vi "P3_2_Complmentos_Simulacion.vi"() -> ()   [LabVIEW 2020]
panel:
  out "consumo de lecha para chocomilk":dynamicdata(graph)
  out "m3 de leche":dbl(knob) scale=0.0..20.0
  out "valor maximo":i32
  out "dato ultimo de leche":i32
  out "calcetoce":dbl(slide) caption="Agua" scale=0.0..20.0
  out "procesos":i32
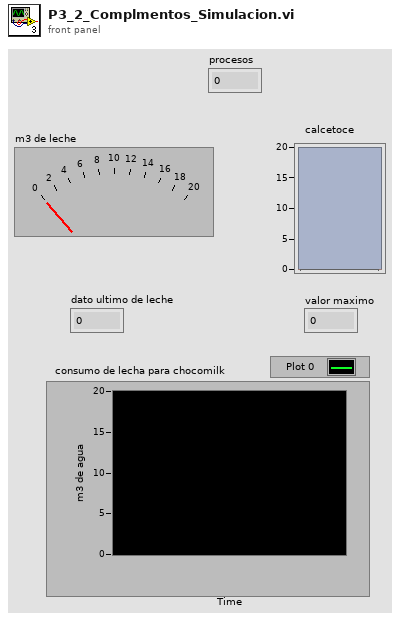
[diagram p1: front panel]
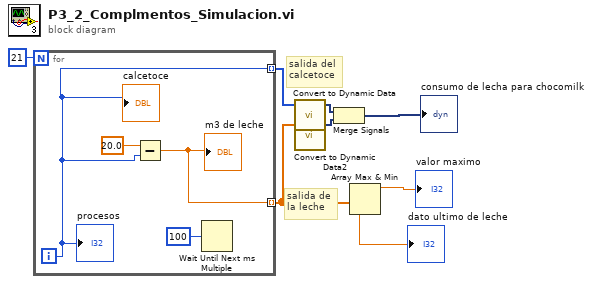
[diagram p0: block diagram]
diagram:
  # "salida del \ncalcetoce"
  # "salida de \nla leche"
  n1 = for {
    N: 21 -> [_]
    tunnel: [w11] -> w2 mode=indexing
    tunnel: [w10] -> w5 mode=indexing
    i -> [w11]
    n2 = Subtract(x=20.0, y=w11) -> (x-y=w10:dbl)
    "m3 de leche" <- w10
    n3 = Wait Until Next ms Multiple(millisecond multiple=100) -> ()  [unwired: 1 out]
    "procesos" <- w11
    "calcetoce" <- w11
  }
  n4 = call "Convert to Dynamic Data"("Array"=w2) -> ("Dynamic Data Type"=w7:dynamicdata)  [unwired: 3 in]
  n5 = call "Convert to Dynamic Data2"("Array"=w5) -> ("Dynamic Data Type"=w6:dynamicdata)  [unwired: 3 in]
  n6 = Merge Signals "Merge Signals"(w7, w6) -> (→"consumo de lecha para chocomilk":dynamicdata)
  n7 = Array Max & Min(array=w5) -> (max value=→"valor maximo":dbl, min value=→"dato ultimo de leche":dbl)  [unwired: 2 out]
